vi "3ph Power Raw to TDMS.vi"(7 "PowRaw Name":string, 9 "Channel Units":string[](array[string])=["V", "V", "V", "A", "A", "A", "UTC"], 10 "Channel Names":string[](array[string])=["MODAQ_Va", "MODAQ_Vb", "MODAQ_Vc", "MODAQ_Ia", "MODAQ_Ib", "MODAQ_Ic", "Time"], 11 "Queue in wfm":refnum<queue>) -> ()   [LabVIEW 2019]
uses:
  Globals and Definitions/Initialization Globals.vi
  Globals and Definitions/RT Globals RD v1.0.vi
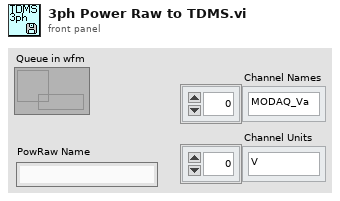
[diagram p1: front panel]
types:
  T1 = typedef "Enum_FileNewInterval.ctl" = enum16{"10 Min", "Hourly", "Daily", "Weekly", "Monthly"}
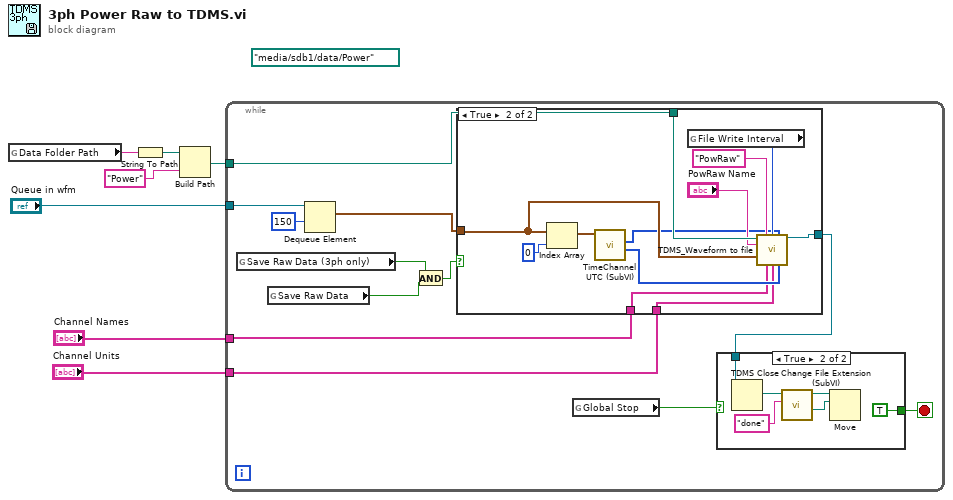
[diagram p0: block diagram]
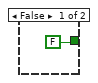
[diagram p2: hidden frame]
diagram:
  (unwired) path "/media/sdb1/data/Power" ("base path")
  n1 = global read "Initialization Globals.vi" "Data Folder Path"() -> (w3:string)
  n2 = String To Path(string=w3) -> (path=w4:path)
  n3 = Build Path(base path=w4, name or relative path="Power") -> (appended path=w2:path)
  n4 = while {
    tunnel: "Channel Names" -> [w16]
    tunnel: "Channel Units" -> [w19]
    tunnel: w2 -> [w15]
    tunnel: "Queue in wfm" -> [w10]
    stop <- w17 stop-if-true
    n5 = global read "Initialization Globals.vi" "Save Raw Data (3ph only)"() -> (w13:bool)
    n6 = global read "Initialization Globals.vi" "Save Raw Data"() -> (w12:bool)
    n7 = Dequeue Element(queue=w10, timeout in ms (-1)=150) -> (element=w9:waveform(dbl)[])  [unwired: 1 in, 3 out]
    n8 = And(x=w13, y=w12) -> (x .and. y?=w14:bool)
    n9 = case shown="True" w14 {
      tunnel: w15 -> [_ w33]
      tunnel: w9 -> [_ w30]
      tunnel: w16 -> [_ w34]
      tunnel: w19 -> [_ w35]
      tunnel: [_ w31] -> w18
      frame False {
      }
      frame True {
        n10 = Index Array(array=w30, index=0) -> (element=w37:waveform(dbl))
        n11 = call "TimeChannel UTC (SubVI).vi"("Waveform"=w37) -> ("UTC Time SC DAQmx"=w36:u64[], "UTC Time FPGA"=w27:u64[])  [unwired: 8 in, 1 out]
        n12 = global read "Initialization Globals.vi" "File Write Interval"() -> (w28:T1)
        n13 = call "TDMS_Waveform to file.vi"("Base path"=w33, "Group Name"="PowRaw", "Interval"=w28, "UTC Time FPGA"=w27, "Measurement"="PowRaw Name", "element"=w30, "Channel Names"=w34, "property values"=w35, "UTC Time SC"=w36) -> ("file out"=w31:refnum<k34>)  [unwired: 5 in, 1 out]
      }
    }
    n14 = global read "RT Globals RD v1.0.vi" "Global Stop"() -> (w11:bool)
    n15 = case shown="True" w11 {
      tunnel: [FALSE TRUE] -> w17
      tunnel: w18 -> [_ w25]
      frame False {
      }
      frame True {
        n16 = TDMS Close(11:w25) -> (3:w24:path)  [unwired: 1 in, 1 out]
        n17 = call "Change File Extension (SubVI).vi"("New Extension"="done", "appended path"=w24) -> ("New file path"=w21:path, "Original Path"=w22:path)  [unwired: 7 in, 1 out]
        n18 = Move(source path=w22, 10:w21) -> ()  [unwired: 3 in, 3 out]
      }
    }
  }
